vi "Acquire_Image_Diff.vi"(11 "CameraDevRef":T1) -> ()   [LabVIEW 2012]
uses:
  <vilib>/Rock Robotics/WPI/Camera/WPI_CameraDevRef.ctl
  <vilib>/vision/NI_Vision_Development_Module.lvlib
panel:
  in  "Threshold Range":cluster{"Lower value":sgl, "Upper value":sgl}={"Lower value"=200.0, "Upper value"=255.0} {"Upper value" format="%.2f"; "Lower value" format="%.2f"}
  out "Light Image Out":T2(plugin-control)
  out "Dark Image Out":T2(plugin-control)
  out "Light Green Image Out":T2(plugin-control)
  out "Dark Green Image Out":T2(plugin-control)
  out "Difference":T2(plugin-control)
  out "Dark Binary":T2(plugin-control)
  out "Light Binary":T2(plugin-control)
  out "dt take":u32
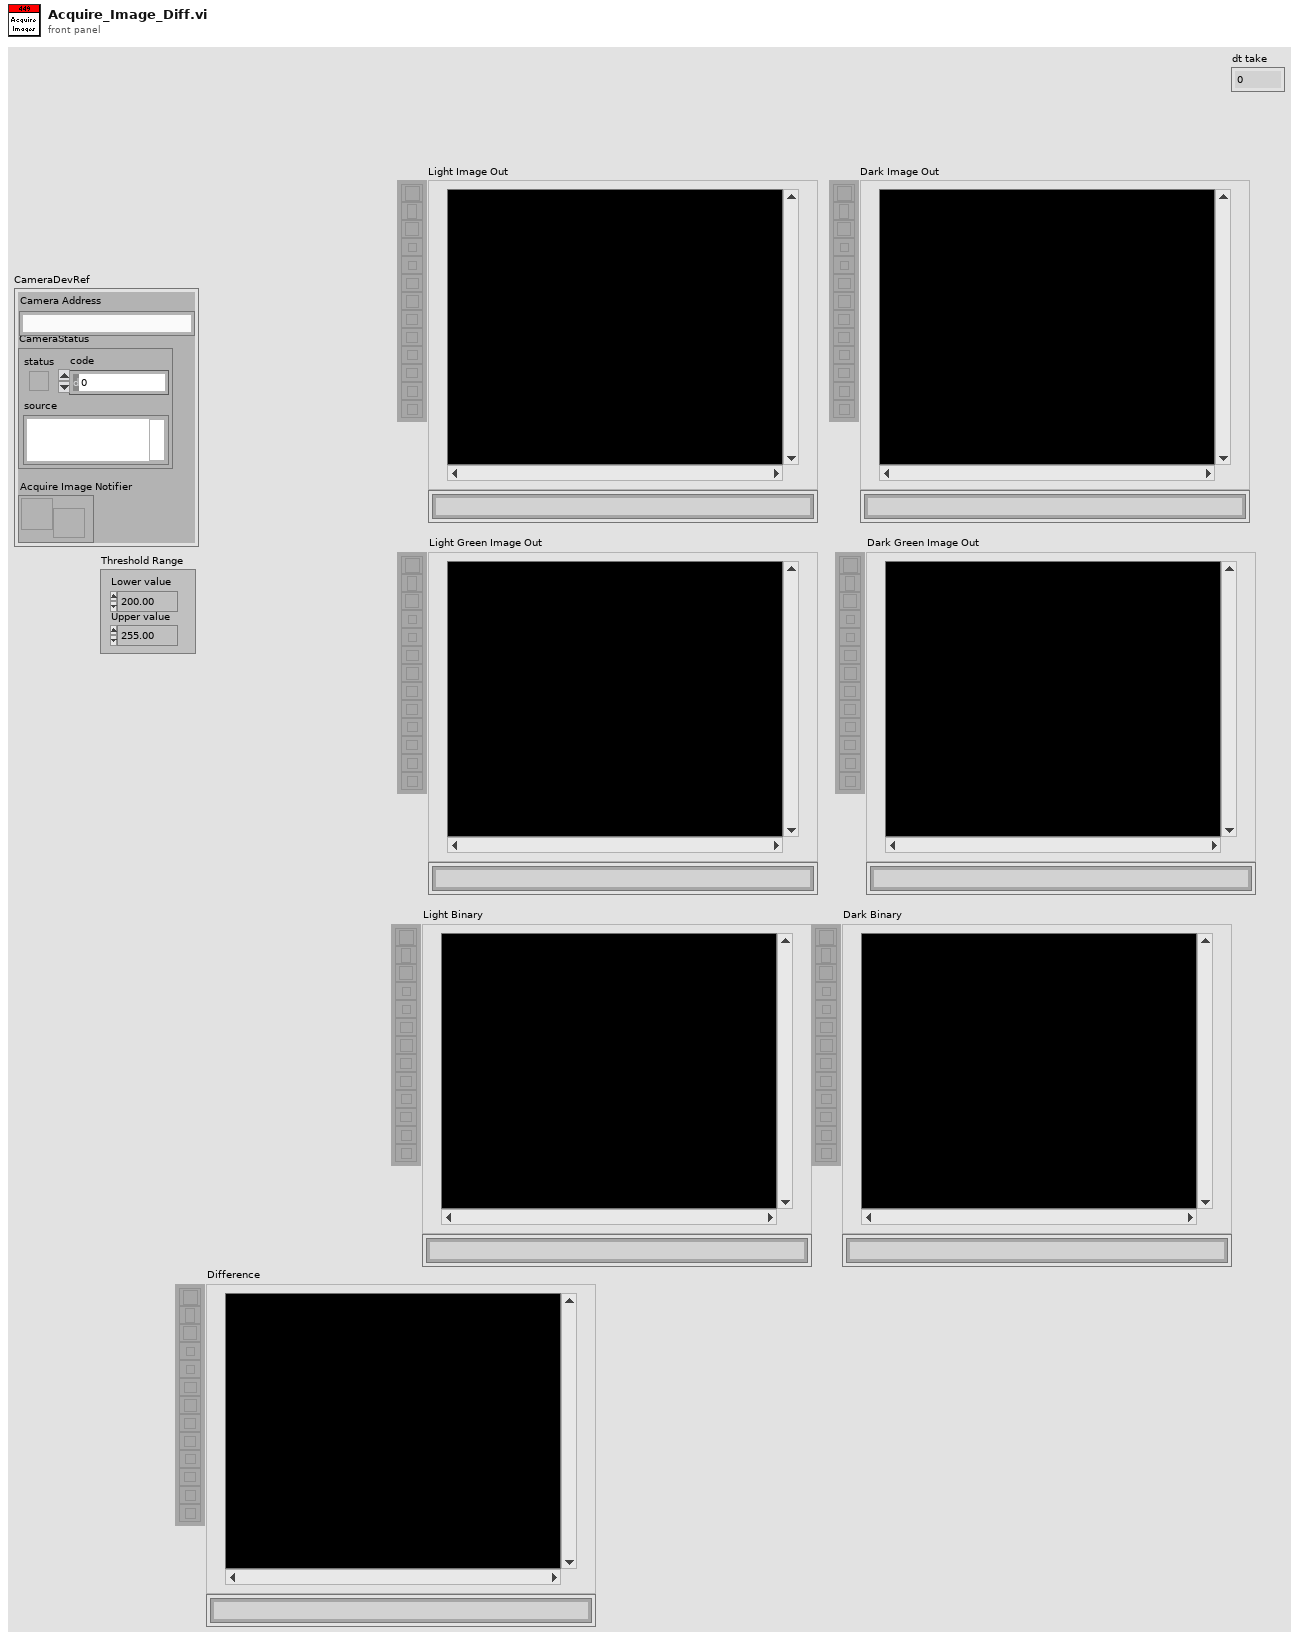
[diagram p1: front panel]
types:
  T1 = typedef "WPI_CameraDevRef.ctl" = cluster{"Camera Address":string, "CameraStatus":errorcluster, "Acquire Image Notifier":refnum<notifier>}
  T2 = typedef "IMAQ Image.ctl" = refnum<image>
  T3 = typedef "Image Cluster.ctl" = cluster{"Input Image Light":T2, "Input Image Dark":T2, "Rotated Image Light":T2, "Rotated Image Dark":T2, "Green Image Light":T2, "Green Image Dark":T2, "Binary Image Light":T2, "Binary Difference":T2, "Binary Image Dark":T2, "Final Binary":T2, "Horizontal Calibration":T2}
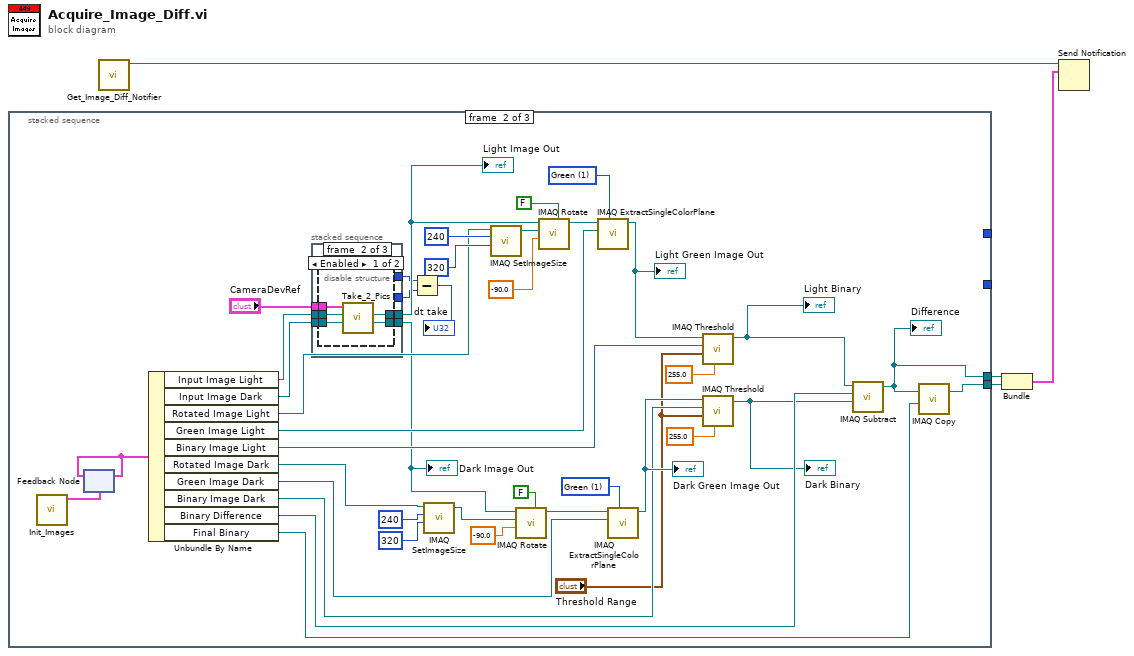
[diagram p0: block diagram]
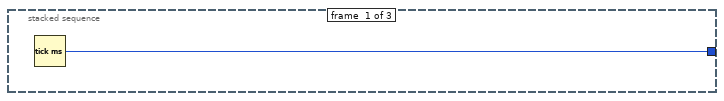
[diagram p2: hidden frame]
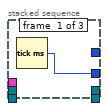
[diagram p3: hidden frame]
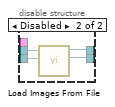
[diagram p4: hidden frame]
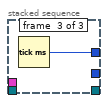
[diagram p5: hidden frame]
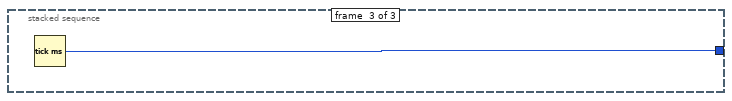
[diagram p6: hidden frame]
diagram:
  n1 = stacked-sequence {
    tunnel: [_ w14 _] -> w2
    tunnel: [_ w13 _] -> w3
    tunnel: [w5 _ _] -> _
    tunnel: [_ _ w63] -> _
    frame #0 {
      n2 = Tick Count (ms)() -> (millisecond timer value=w5:u32)
    }
    frame #1 {
      w35 = 1 items=["Red", "Green", "Blue", "Hue", "Saturation", "Luminance", "Value", "Intensity"] ("Color Plane")
      w38 = 1 items=["Red", "Green", "Blue", "Hue", "Saturation", "Luminance", "Value", "Intensity"] ("Color Plane")
      n3 = call "Init_Images.vi"() -> ("Images"=w34:T3)  [unwired: 11 in]
      n4 = feedback #1(w34) -> (w33:T3)
      n5 = feedback-in #1(w33) -> ()
      n6 = Unbundle By Name(w33) -> ("Input Image Light"=w32:T2, "Input Image Dark"=w31:T2, "Rotated Image Light"=w30:T2, "Green Image Light"=w28:T2, "Binary Image Light"=w21:T2, "Rotated Image Dark"=w27:T2, "Green Image Dark"=w26:T2, "Binary Image Dark"=w23:T2, "Binary Difference"=w19:T2, "Final Binary"=w16:T2)
      n7 = stacked-sequence {
        tunnel: "CameraDevRef" -> [_ w52 _]
        tunnel: w32 -> [_ w51 _]
        tunnel: w31 -> [_ w50 _]
        tunnel: [_ w49 _] -> w29
        tunnel: [_ w48 _] -> w15
        tunnel: [w47 _ _] -> w12
        tunnel: [_ _ w62] -> w11
        frame #0 {
          n8 = Tick Count (ms)() -> (millisecond timer value=w47:u32)
        }
        frame #1 {
          n9 = disable-structure shown="Enabled" {
            disable-tunnel: w52 -> [w57 _]
            disable-tunnel: w51 -> [w56 w59]
            disable-tunnel: w50 -> [w55 w58]
            disable-tunnel: [w54 w61] -> w49
            disable-tunnel: [w53 w60] -> w48
            frame Enabled {
              n10 = call "Take_2_Pics.vi"("Image Src Dark"=w55, "Image Src Light"=w56, "CameraDevRef"=w57) -> ("Image Out Dark"=w53:T2, "Image Out Light"=w54:T2)  [unwired: 7 in]
            }
            frame Disabled {
              n11 = call "Load Images From File.vi"("Input Image Dark"=w58, "Input Image Light"=w59) -> ("Dark Image Out"=w60:T2, "Light Image Out"=w61:T2)  [unwired: 8 in]
            }
          }
        }
        frame #2 {
          n12 = Tick Count (ms)() -> (millisecond timer value=w62:u32)
        }
      }
      "Light Image Out" <- w29
      "Dark Image Out" <- w15
      n13 = Subtract(x=w11, y=w12) -> (x-y=→"dt take":u32)
      n14 = call "IMAQ SetImageSize"("Y Resolution"=320 ("X Resolution"), "X Resolution"=240 ("Y Resolution"), "Image"=w27) -> ("Image Out"=w44:T2)  [unwired: 2 in, 1 out]
      n15 = call "IMAQ SetImageSize"("Y Resolution"=320 ("X Resolution"), "X Resolution"=240 ("Y Resolution"), "Image"=w30) -> ("Image Out"=w8:T2)  [unwired: 2 in, 1 out]
      n16 = call "IMAQ Rotate"("Maintain Size"=FALSE, "Angle (degrees)"=sgl -90.0, "Image Dst"=w44, "Image Src"=w15) -> ("Image Dst Out"=w37:T2)  [unwired: 6 in, 1 out]
      n17 = call "IMAQ Rotate"("Maintain Size"=FALSE, "Angle (degrees)"=sgl -90.0, "Image Dst"=w8, "Image Src"=w29) -> ("Image Dst Out"=w36:T2)  [unwired: 6 in, 1 out]
      n18 = call "IMAQ ExtractSingleColorPlane"("Color Plane"=w35, "Image Dst"=w28, "Image Src"=w36) -> ("Image Dst Out"=w22:T2)  [unwired: 7 in, 1 out]
      "Light Green Image Out" <- w22
      n19 = call "IMAQ ExtractSingleColorPlane"("Color Plane"=w38, "Image Dst"=w26, "Image Src"=w37) -> ("Image Dst Out"=w24:T2)  [unwired: 7 in, 1 out]
      "Dark Green Image Out" <- w24
      n20 = call "IMAQ Threshold"("Replace Value"=sgl 255.0, "Range"="Threshold Range", "Image Dst"=w21, "Image Src"=w22) -> ("Image Dst Out"=w17:T2)  [unwired: 6 in, 1 out]
      "Light Binary" <- w17
      n21 = call "IMAQ Threshold"("Replace Value"=sgl 255.0, "Range"="Threshold Range", "Image Dst"=w23, "Image Src"=w24) -> ("Image Dst Out"=w18:T2)  [unwired: 6 in, 1 out]
      "Dark Binary" <- w18
      n22 = call "IMAQ Subtract"("Image Src A"=w17, "Image Dst"=w19, "Image Src B"=w18) -> ("Image Dst Out"=w13:T2)  [unwired: 4 in, 1 out]
      "Difference" <- w13
      n23 = call "IMAQ Copy"("Image Dst"=w16, "Image Src"=w13) -> ("Image Dst Out"=w14:T2)  [unwired: 4 in, 1 out]
    }
    frame #2 {
      n24 = Tick Count (ms)() -> (millisecond timer value=w63:u32)
    }
  }
  n25 = call "Get_Image_Diff_Notifier.vi"() -> ("notifier out"=w4:refnum<notifier>)  [unwired: 11 in]
  n26 = Bundle("Image Dst Out"=w3, "Image Dst Out"=w2) -> (w1:cluster{"Image Dst Out":T2, "Image Dst Out":T2})  [unwired: 1 in]
  n27 = Send Notification(notification=w1, notifier=w4) -> ()  [unwired: 1 in, 2 out]
